vi "Log Testing.vi"() -> ()   [LabVIEW 2012]
uses:
  Logging VIs/Log Entry Block.ctl
  Logging VIs/Log Entry.ctl
  Logging VIs/Log Value Type.ctl
  Logging VIs/Log Value Cluster.ctl
  Logging VIs/Logging Equals - Entries.vi
  Logging VIs/Logging Update - Boolean.vi
  Logging VIs/Logging Update - Numeric.vi
  femtoRoboLib.lvlib
panel:
  out "Numeric":dbl
  in  "Scrollbar":u32(c297)
  in  "Stop":bool=TRUE
  out "Tree":string(tree)
  out "Times":u32[](array[numeric])
  out "Log":T1[](array[typedef])
  out "Output":T1
  in  "Write":bool
  in  "/pie/llama":dbl
  in  "/moo/num":dbl
  in  "/moo/bool":bool
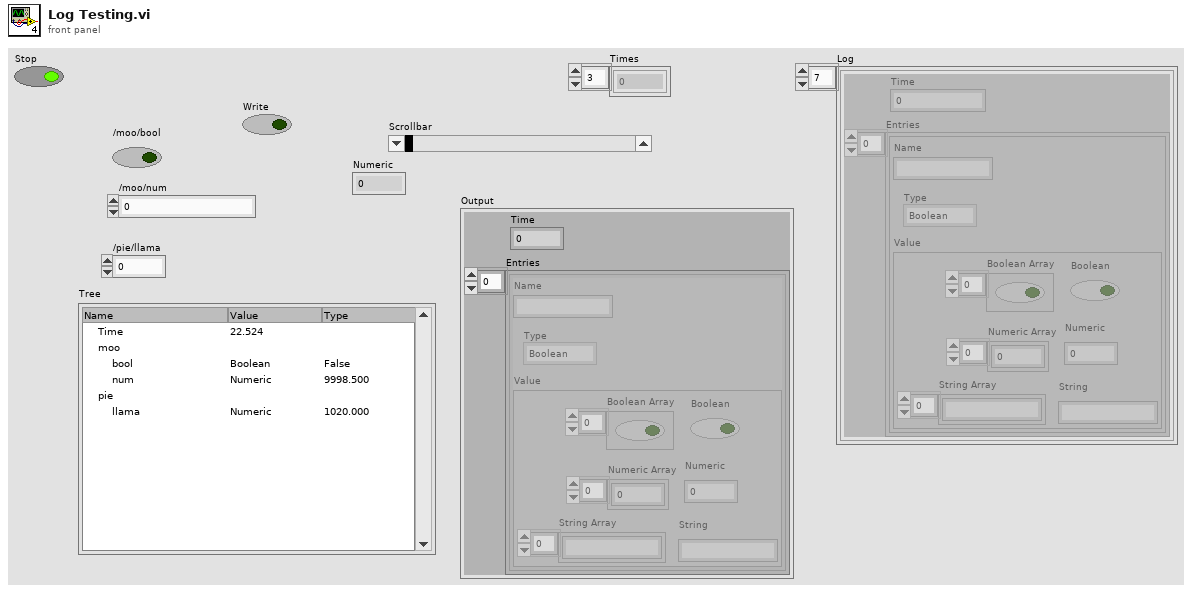
[diagram p1: front panel]
types:
  T1 = typedef "femtoRoboLib.lvlib/Log Entry Block.ctl" = cluster{"Entries":T2[], "Time":u32}
  T2 = typedef "femtoRoboLib.lvlib/Log Entry.ctl" = cluster{"Name":string, "Type":T3, "Value":T4}
  T3 = typedef "femtoRoboLib.lvlib/Log Value Type.ctl" = enum16{"Boolean", "Numeric", "String", "Boolean Array", "Numeric Array", "String Array"}
  T4 = typedef "femtoRoboLib.lvlib/Log Value Cluster.ctl" = cluster{"Boolean Array":bool[], "Boolean":bool, "Numeric Array":dbl[], "Numeric":dbl, "String Array":string[], "String":string}
  T5 = typedef "femtoRoboLib.lvlib/LoggingDevRef.ctl" = cluster{"DevStatus":errorcluster, "refnum":refnum<file>, "Path":path, "Start Time":u32}
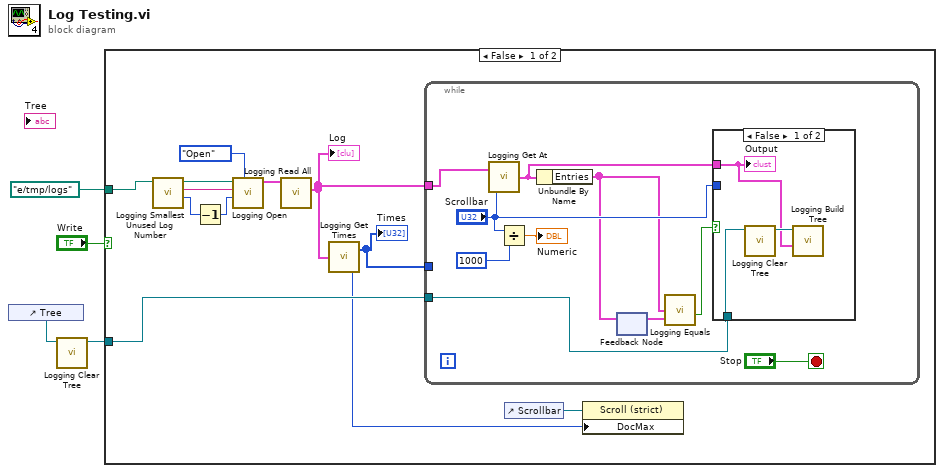
[diagram p0: block diagram]
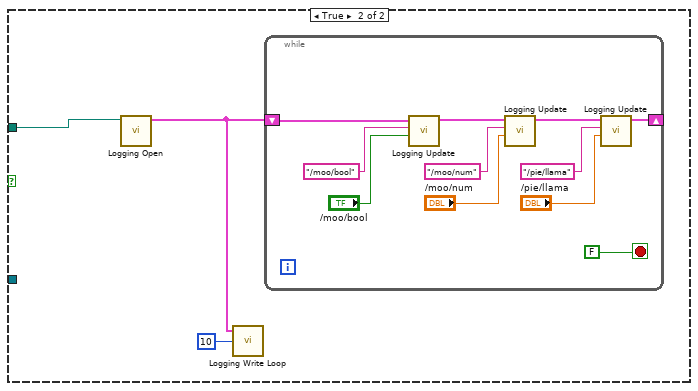
[diagram p3: hidden frame]
diagram:
  n1 = control-ref of="Tree"() -> (w2:refnum<vi>)
  n2 = call "Logging Clear Tree.vi"("TreeRef"=w2) -> ("TreeRef"=w1:refnum<vi>)  [unwired: 6 in]
  n3 = case shown="False" "Write" {
    tunnel: path "e:/tmp/logs" ("base path") -> [w11 w32]
    tunnel: w1 -> [w15 _]
    frame False {
      n4 = call "Logging Smallest Unused Log Number.vi"("base path"=w11) -> ("Number"=w5:i32, "name out"=w9:string, "base path out"=w10:path)  [unwired: 7 in, 1 out]
      n5 = Decrement(x=w5) -> (x-1=w6:i32)
      n6 = call "Logging Open.vi"("Mode"=enum16{"Create", "Open"}."Open", "Number"=w6, "name"=w9, "base path"=w10) -> ("LoggingDevRef"=w7:T5)  [unwired: 5 in, 1 out]
      n7 = call "Logging Read All.vi"("LoggingDevRef"=w7) -> ("Log"=w16:T1[])  [unwired: 4 in, 2 out]
      "Log" <- w16
      n8 = call "Logging Get Times.vi"("Log Input"=w16) -> ("Times"=w14:u32[], "Latest"=w12:u32)
      "Times" <- w14
      n9 = while {
        tunnel: w16 -> [w22]
        tunnel: w15 -> [w26]
        tunnel: w14 -> [_]
        stop <- "Stop" stop-if-true
        n10 = call "Logging Get At.vi"("Time (ms)"="Scrollbar", "Log Input"=w22) -> ("Output"=w18:T1)
        n11 = Divide(x="Scrollbar", y=u32 1000) -> (x/y=→"Numeric":dbl)
        n12 = Unbundle By Name(w18) -> ("Entries"=w17:T2[])
        n13 = feedback-in #1(w17) -> ()
        n14 = feedback #1() -> (w20:T2[])  [unwired: 1 in]
        n15 = call-poly "Logging Equals.vi"("Entries A"=w17, "Entries B"=w20) -> ("Equal"=w19:bool)  [unwired: 4 in]
        n16 = case shown="False" w19 {
          tunnel: w26 -> [w28 _]
          tunnel: "Scrollbar" -> [_ _]
          tunnel: w18 -> [w27 _]
          frame False {
            n17 = call "Logging Clear Tree.vi"("TreeRef"=w28) -> ("TreeRef"=w29:refnum<vi>)  [unwired: 6 in]
            n18 = call "Logging Build Tree.vi"("Entries"=w27, "TreeRef"=w29) -> ()  [unwired: 5 in, 1 out]
            "Output" <- w27
          }
          frame True {
          }
        }
      }
      n19 = control-ref of="Scrollbar"() -> (w13:refnum<vi>)
      n20 = property class="Scroll (strict)"(reference=w13, "DocMax"=w12) -> ()  [unwired: 1 in, 2 out]
    }
    frame True {
      n21 = call "Logging Open.vi"("base path"=w32) -> ("LoggingDevRef"=w30:T5)  [unwired: 8 in, 1 out]
      n22 = call "Logging Write Loop.vi"("Delay"=u32 10, "LoggingDevRef"=w30) -> ()  [unwired: 4 in]
      n23 = while {
        shift-right: [w36] -> _
        shift-left: w30 -> [w41]
        stop <- FALSE stop-if-true
        n24 = call-poly "Logging Update.vi"("Value"="/moo/bool", "Name"="/moo/bool", "LoggingDevRef"=w41) -> ("LoggingDevRef"=w39:T5)  [unwired: 3 in, 1 out]
        n25 = call-poly "Logging Update.vi"("Value"="/moo/num", "Name"="/moo/num", "LoggingDevRef"=w39) -> ("LoggingDevRef"=w37:T5)  [unwired: 3 in, 1 out]
        n26 = call-poly "Logging Update.vi"("Value"="/pie/llama", "Name"="/pie/llama", "LoggingDevRef"=w37) -> ("LoggingDevRef"=w36:T5)  [unwired: 3 in, 1 out]
      }
    }
  }
